vi "H1R Heuristic.vi"() -> ()   [LabVIEW 2013, in "Scheduler.lvclass"]
uses:
  Scheduler.lvclass
panel:
  out "Lower Bound":u16
  out "Start Times":u16[][](array[numeric])
  out "Schedule Order":u16[](array[numeric])
  out "Schedule":u16[](array[numeric])
  out "Machine Completion Time":u16[](array[numeric])
  out "Job Completion Times":u16[](array[numeric])
  out "Completion Times":u16[][](array[numeric])
  in  "Number of  Jobs":i32=4
  in  "Number of Machines":i32=4
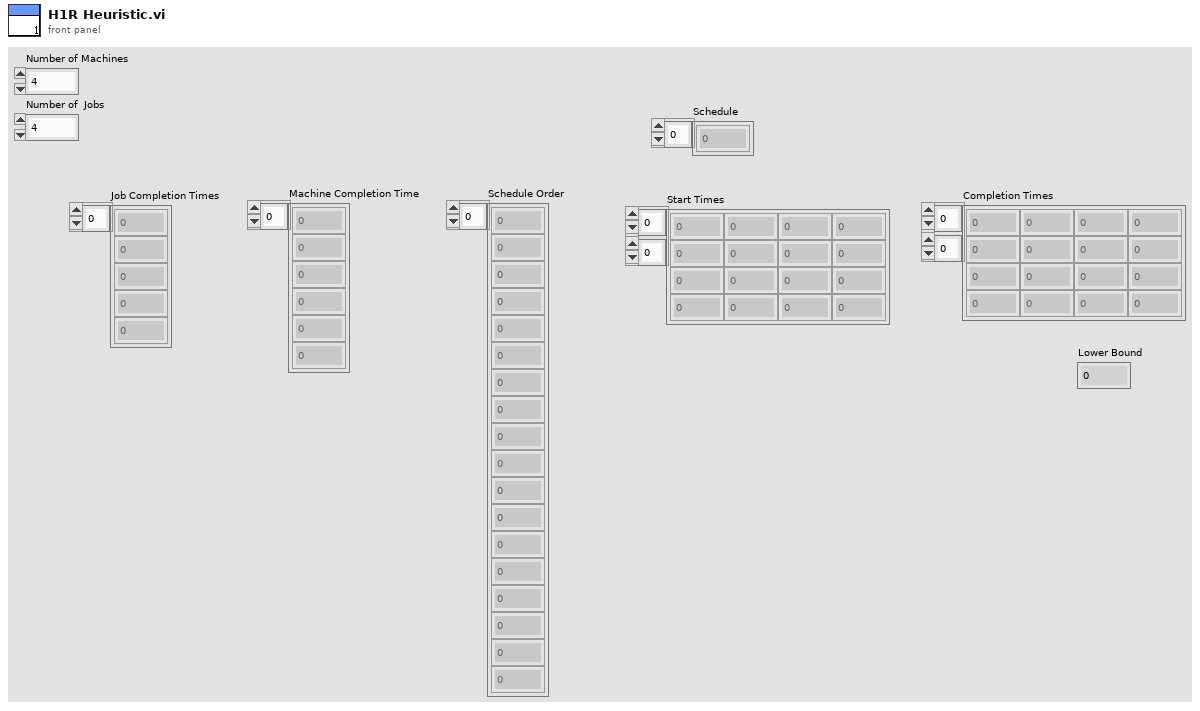
[diagram p1: front panel]
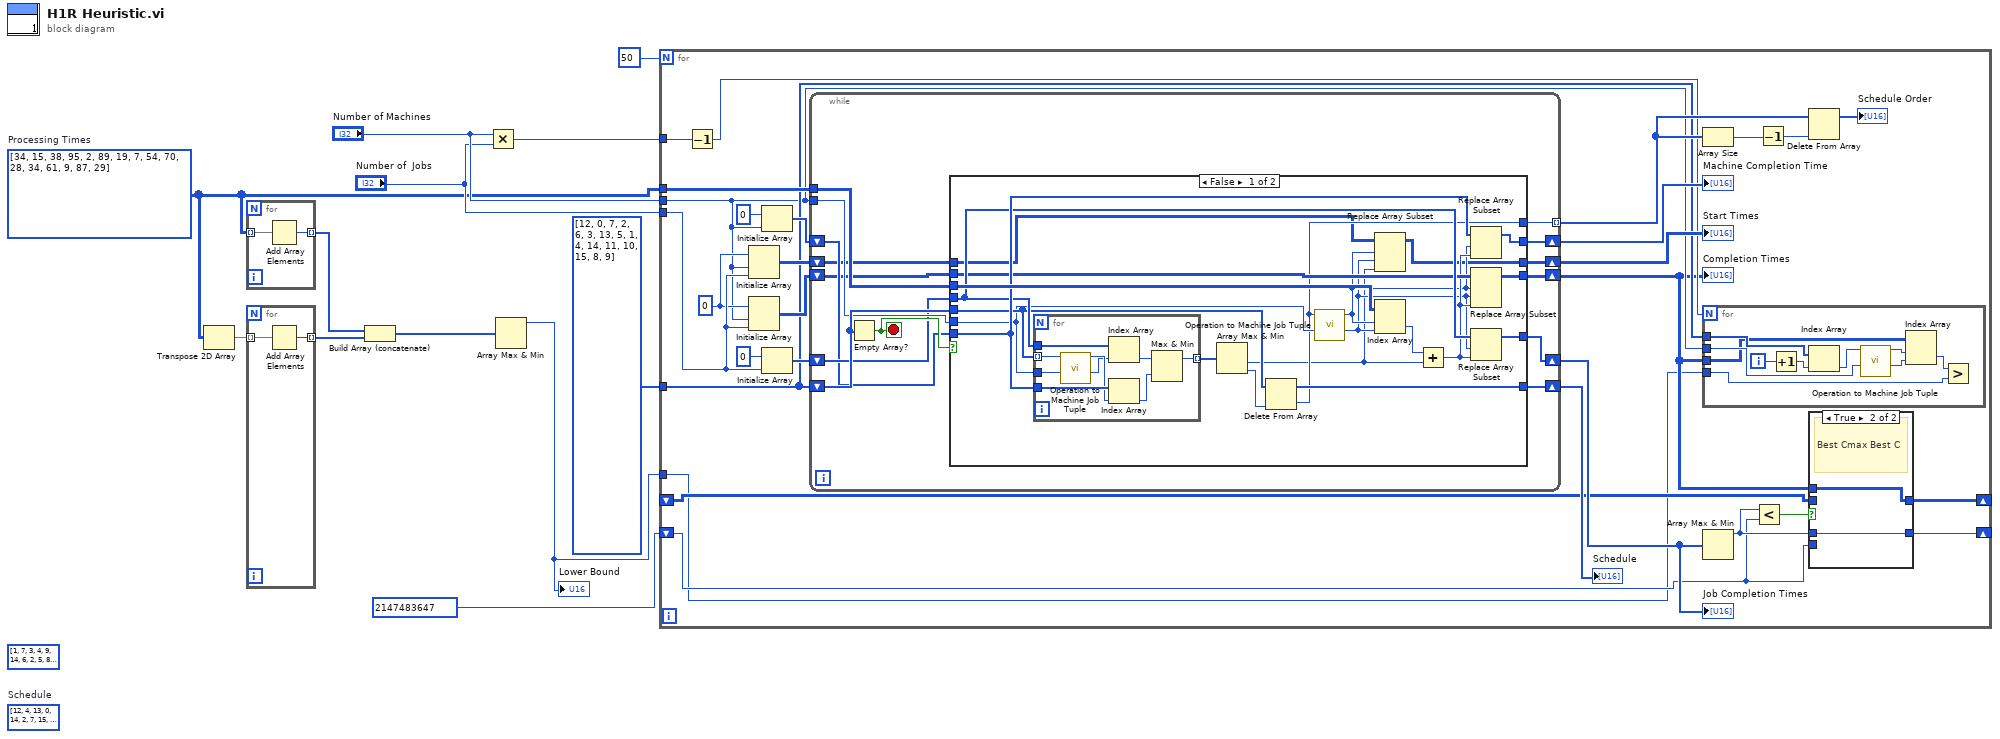
[diagram p0: block diagram]
diagram:
  (unwired) u16[] [1, 7, 3, 4, 9, 14, 6, 2, 5, 8, 13, 11, 0, 12, 10, 15] ("Schedule")
  w6 = u16[][] [[34, 15, 38, 95], [2, 89, 19, 7], [54, 70, 28, 34], [61, 9, 87, 29]]  # Processing Times
  (unwired) u16[] [12, 4, 13, 0, 14, 2, 7, 15, 9, 1, 6, 3, 11, 10, 5, 8]  # Schedule
  n1 = Transpose 2D Array(2D array=w6) -> (transposed array=w5:u16[][])
  n2 = for {
    tunnel: w6 -> [w14] mode=indexing
    tunnel: [w13] -> w4 mode=indexing
    n3 = Add Array Elements(numeric array=w14) -> (sum=w13:u16)
  }
  n4 = for {
    tunnel: w5 -> [w16] mode=indexing
    tunnel: [w15] -> w3 mode=indexing
    n5 = Add Array Elements(numeric array=w16) -> (sum=w15:u16)
  }
  n6 = Build Array (concatenate)(w4, w3) -> (w2:u16[])
  n7 = Multiply(x="Number of Machines", y="Number of  Jobs") -> (x*y=w7:i32)
  n8 = Array Max & Min(array=w2) -> (max value=w1:u16)  [unwired: 3 out]
  "Lower Bound" <- w1
  n9 = for {
    N: 50 -> [_]
    tunnel: w6 -> [w41]
    tunnel: "Number of Machines" -> [w19]
    tunnel: "Number of  Jobs" -> [w33]
    shift-right: [w27] -> _
    shift-left: 2147483647 -> [w25]
    tunnel: u16[] [12, 0, 7, 2, 6, 3, 13, 5, 1, 4, 14, 11, 10, 15, 8, 9] -> [w22]
    shift-right: [w24] -> _
    shift-left: _ -> [w23]
    tunnel: w7 -> [w21]
    tunnel: w1 -> [w17]
    w32 = u16 0 ("element")
    n10 = Decrement(x=w21) -> (x-1=w20:i32)
    n11 = Initialize Array(w32, w19, w33) -> (w31:u16[][])
    n12 = Initialize Array(w32, w19, w33) -> (w40:u16[][])
    n13 = Initialize Array(u16 0 ("element"), w19) -> (w42:u16[])
    n14 = Initialize Array(u16 0 ("element"), w33) -> (w43:u16[])
    n15 = while {
      shift-right: [w65] -> w38
      shift-left: w22 -> [w72]
      tunnel: w19 -> [w71]
      shift-right: [w68] -> w29
      shift-left: w43 -> [w70]
      shift-right: [w67] -> w39
      shift-left: w42 -> [w69]
      shift-right: [w63] -> w18
      shift-left: w40 -> [w64]
      tunnel: w41 -> [w66]
      tunnel: [w62] -> w37 mode=indexing
      shift-right: [w60] -> w30
      shift-left: w31 -> [w61]
      stop <- w73 stop-if-true
      n16 = Empty Array?(array=w72) -> (empty?=w73:bool)
      n17 = case shown="False" w73 {
        tunnel: w72 -> [w85 w105]
        tunnel: w71 -> [w80 _]
        tunnel: w70 -> [w91 w107]
        tunnel: w69 -> [w92 w106]
        tunnel: [w90 w107] -> w68
        tunnel: [w89 w106] -> w67
        tunnel: w66 -> [w93 _]
        tunnel: [w84 w105] -> w65
        tunnel: w64 -> [w88 w104]
        tunnel: [w87 w104] -> w63
        tunnel: [w79 _] -> w62
        tunnel: w61 -> [w78 w103]
        tunnel: [w74 w103] -> w60
        frame False {
          n18 = for {
            tunnel: w85 -> [w102] mode=indexing
            tunnel: w80 -> [w101]
            tunnel: w91 -> [w98]
            tunnel: w92 -> [w100]
            tunnel: [w94] -> w86 mode=indexing
            n19 = call "Operation to Machine Job Tuple.vi"("Number of Machines"=w101, "Operation Number"=w102) -> ("Job No"=w97:i32, "Machine No"=w99:i32)  [unwired: 8 in]
            n20 = Index Array(array=w98, index=w97) -> (element=w96:u16)
            n21 = Index Array(array=w100, index=w99) -> (element=w95:u16)
            n22 = Max & Min(x=w96, y=w95) -> (max(x,y)=w94:u16)  [unwired: 1 out]
          }
          n23 = Array Max & Min(array=w86) -> (min value=w75:u16, min index (indices)=w81:i32)  [unwired: 2 out]
          n24 = Delete From Array(array=w85, index=w81) -> (deleted portion=w79:u16, array with subset deleted=w84:u16[])  [unwired: 1 in]
          n25 = call "Operation to Machine Job Tuple.vi"("Number of Machines"=w80, "Operation Number"=w79) -> ("Job No"=w76:i32, "Machine No"=w77:i32)  [unwired: 8 in]
          n26 = Replace Array Subset(array=w78, new element=w75, index (row)=w77, index (col)=w76) -> (w74:u16[][])
          n27 = Index Array(array=w93, index (row)=w77, index (col)=w76) -> (element=w83:u16)
          n28 = Add(x=w83, y=w75) -> (x+y=w82:u16)
          n29 = Replace Array Subset(array=w92, new element=w82, index=w77) -> (w89:u16[])
          n30 = Replace Array Subset(array=w88, new element=w82, index (row)=w77, index (col)=w76) -> (w87:u16[][])
          n31 = Replace Array Subset(array=w91, new element=w82, index=w76) -> (w90:u16[])
        }
        frame True {
        }
      }
    }
    "Completion Times" <- w18
    "Job Completion Times" <- w29
    "Machine Completion Time" <- w39
    "Schedule" <- w38
    "Start Times" <- w30
    n32 = Array Size(array=w37) -> (size(s)=w36:i32)
    n33 = for {
      N: w20 -> [_]
      tunnel: w22 -> [w55]
      tunnel: w19 -> [w51]
      tunnel: w18 -> [w50]
      tunnel: w17 -> [w46]
      i -> [w54]
      n34 = Increment(x=w54) -> (x+1=w53:i32)
      n35 = Index Array(array=w55, index=w53) -> (element=w52:u16)
      n36 = call "Operation to Machine Job Tuple.vi"("Number of Machines"=w51, "Operation Number"=w52) -> ("Job No"=w48:i32, "Machine No"=w49:i32)  [unwired: 8 in]
      n37 = Index Array(array=w50, index (row)=w49, index (col)=w48) -> (element=w47:u16)
      n38 = Greater?(x=w47, y=w46) -> ()  [unwired: 1 out]
    }
    n39 = Array Max & Min(array=w29) -> (max value=w26:u16)  [unwired: 3 out]
    n40 = Less?(x=w26, y=w25) -> (x < y?=w28:bool)
    n41 = Decrement(x=w36) -> (x-1=w35:i32)
    n42 = Delete From Array(array=w37, index=w35) -> (array with subset deleted=→"Schedule Order":u16[])  [unwired: 1 in, 1 out]
    n43 = case shown="True" w28 {
      tunnel: [w57 w59] -> w27
      tunnel: w26 -> [_ w59]
      tunnel: w25 -> [w57 _]
      tunnel: w18 -> [_ w58]
      tunnel: [w56 w58] -> w24
      tunnel: w23 -> [w56 _]
      frame False {
      }
      frame True {
        # "Best Cmax Best C"
      }
    }
  }
